vi "get channels.vi"(11 "Shared Library Module configuration in":refnum<class "Shared Library Module configuration.lvclass">) -> (2 "channels":refnum<class "TBM channel.lvclass">[](array[class]), 3 "Shared Library Module configuration out":refnum<class "Shared Library Module configuration.lvclass">)   [LabVIEW 2013, in "Shared Library Module configuration.lvclass"]
doc: "Platypus Framework 1.0.1.60\nNI Systems Engineering - National Instruments"
uses:
  Shared Library Module configuration.lvclass
  <vilib>/NI/Tag Bus Module Framework/channel/TBM channel.lvclass
  Shared Library Module configuration.lvclass/Shared Library Module configuration.ctl
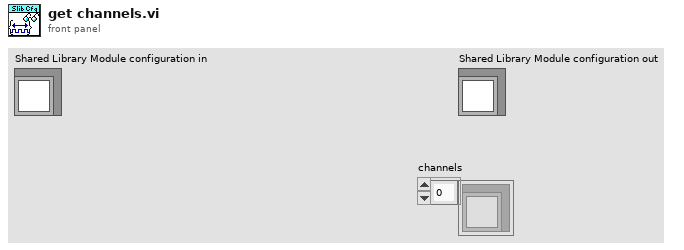
[diagram p1: front panel]
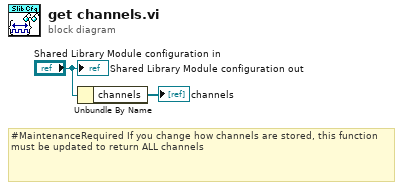
[diagram p0: block diagram]
diagram:
  # "#MaintenanceRequired If you change how channels are stored, this function must be updated to return ALL channels"
  n1 = Unbundle By Name("Shared Library Module configuration in") -> ("channels"=→"channels":refnum<class "TBM channel.lvclass">[])
  "Shared Library Module configuration out" <- "Shared Library Module configuration in"
